vi "Get System Settings.vi"() -> (3 "SystemStartupSettings":T1)   [LabVIEW 2015]
uses:
  Controls/SystemSettings.ctl
  RT Management.lvclass
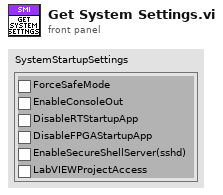
[diagram p1: front panel]
types:
  T1 = typedef "RT Management.lvlib/RT Management.lvclass/SystemSettings.ctl" = cluster{"ForceSafeMode":bool, "EnableConsoleOut":bool, "DisableRTStartupApp":bool, "DisableFPGAStartupApp":bool, "EnableSecureShellServer(sshd)":bool, "LabVIEWProjectAccess":bool}
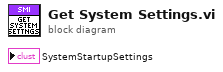
[diagram p0: block diagram]
diagram:
